vi "Flatten path to Filename.vi"(7 "error in (no error)":errorcluster, 9 "Virtual Folder's Virtual Path":string, 10 "Library Base Path":path) -> (0 "error out":errorcluster, 2 "result string":string, 3 "Palette Path":path)   [LabVIEW 2012, in "Palette Generation.lvlib"]
doc: "Takes a virtual folder's virtual path and converts it to a palette file name and palette file real path"
uses:
  Palette Generation.lvlib
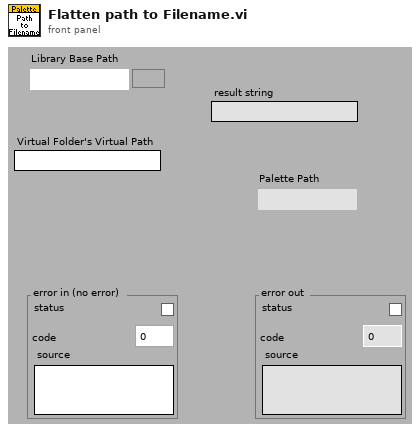
[diagram p1: front panel]
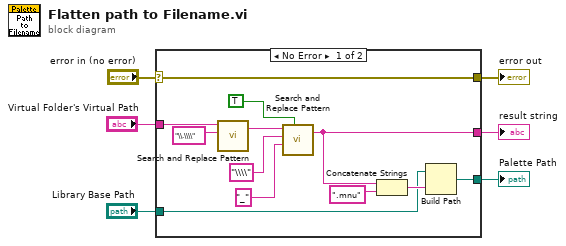
[diagram p0: block diagram]
diagram:
  n1 = case shown="No Error" "error in (no error)" {
    selector: "error in (no error)" -> [w7 w19]
    tunnel: "Virtual Folder's Virtual Path" -> [w13 _]
    tunnel: [w12 _] -> w5
    tunnel: "Library Base Path" -> [w9 _]
    tunnel: [w8 _] -> w3
    tunnel: [w7 w19] -> w2
    frame No Error {
      n2 = call <vilib>:"Search and Replace Pattern.vi"("string"=w13, "regular expression (\"\")"="\\.\\\\" ("regular expression (\"\")")) -> ("result string"=w15:string)  [unwired: 1 in, 3 out]
      n3 = call <vilib>:"Search and Replace Pattern.vi"("string"=w15, "regular expression (\"\")"="\\\\" ("regular expression (\"\")"), "replace string (\"\")"="_" ("replace string (\"\")"), "replace all? (F)"=TRUE) -> ("result string"=w12:string)  [unwired: 2 out]
      n4 = Concatenate Strings(w12, ".mnu" ("string")) -> (w10:string)
      n5 = Build Path(base path=w9, name or relative path=w10) -> (appended path=w8:path)
    }
    frame Error {
    }
  }
  "result string" <- w5
  "Palette Path" <- w3
  "error out" <- w2
